vi "Read Path.vi"(8 "error in (no error)":errorcluster, 11 "Project in":refnum<class "Project.lvclass">) -> (0 "error out":errorcluster, 2 "Path":path, 3 "Project out":refnum<class "Project.lvclass">)   [LabVIEW 2015, in "Project.lvclass"]
uses:
  Project.lvclass
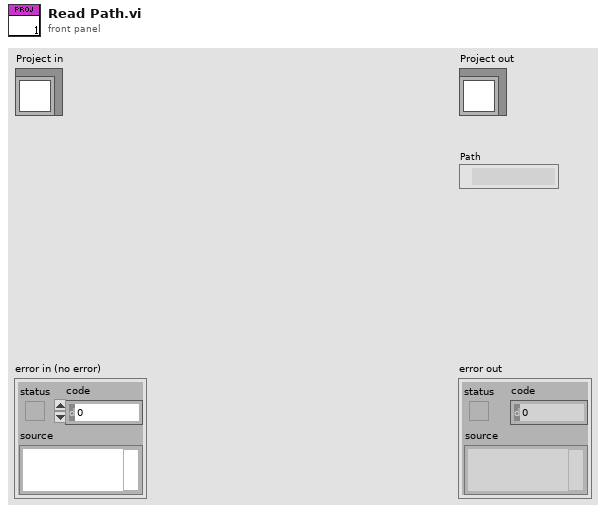
[diagram p1: front panel]
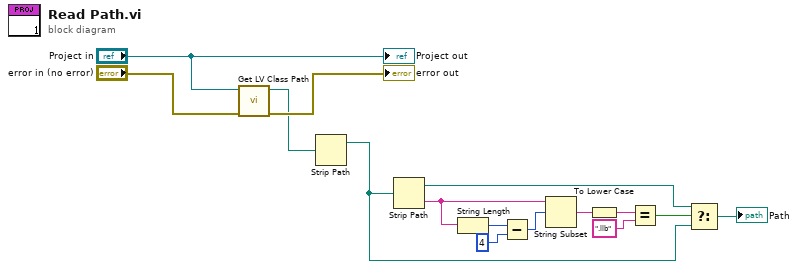
[diagram p0: block diagram]
diagram:
  n1 = call <vilib>:"Get LV Class Path.vi"("error in (no error)"="error in (no error)", "object"="Project in") -> ("error out"=→"error out":errorcluster, "class path"=w2:path)  [unwired: 8 in]
  n2 = Strip Path(path=w2) -> (stripped path=w3:path)  [unwired: 1 out]
  n3 = Strip Path(path=w3) -> (stripped path=w4:path, name=w12:string)
  n4 = String Length(string=w12) -> (length=w11:i32)
  n5 = Subtract(x=w11, y=4) -> (x-y=w9:i32)
  n6 = String Subset(string=w12, offset (0)=w9) -> (substring=w8:string)  [unwired: 1 in]
  n7 = To Lower Case(string=w8) -> (all lower case string=w7:string)
  n8 = Equal?(x=w7, y=".llb") -> (x = y?=w5:bool)
  n9 = Select(t=w4, s=w5, f=w3) -> (s? t:f=→"Path":path)
  "Project out" <- "Project in"
